vi "time wait.vi"(8 "errorIn":errorcluster, 10 "delay(s)":u32=2000, 11 "Mode?":enum16{"Light Mode", "Dark Mode"}(ring)) -> (0 "errorOut":errorcluster)   [LabVIEW 2020]
panel:
  out "Time Remaining":string="   PLEASE WAITING..."
  in  "退出":bool
  out "Cancel?":bool=TRUE
  out "Wait":string="   PLEASE WAITING..."
  out "Slide":i32(slide) scale=0.0..1800000.0
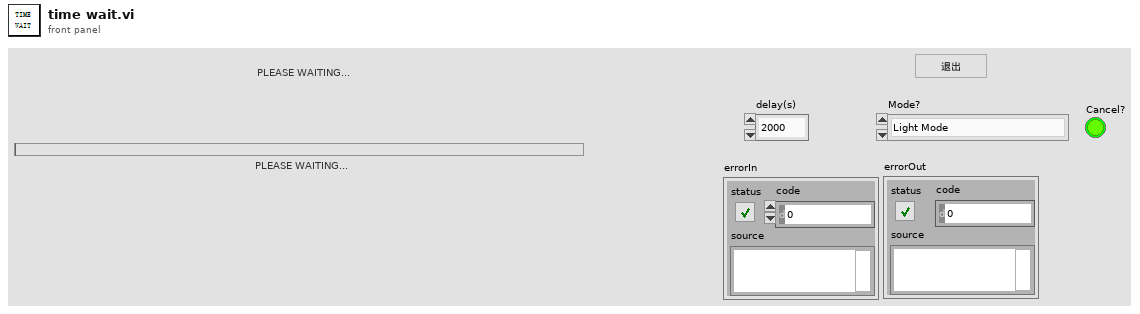
[diagram p1: front panel]
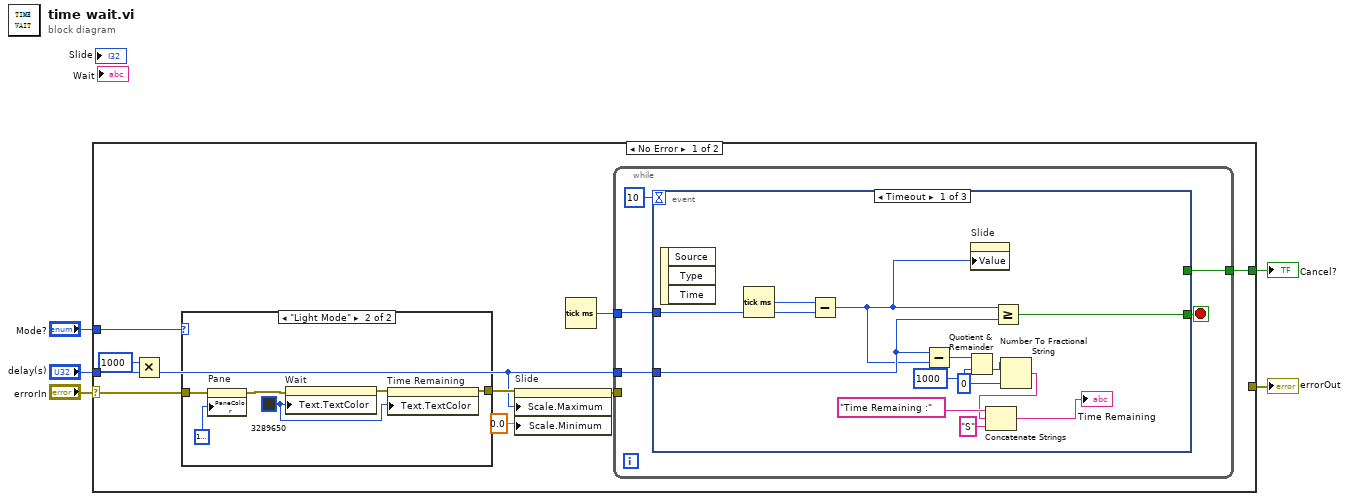
[diagram p0: block diagram]
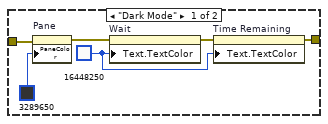
[diagram p2: hidden frame]
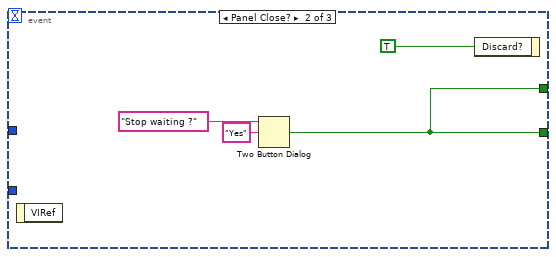
[diagram p3: hidden frame]
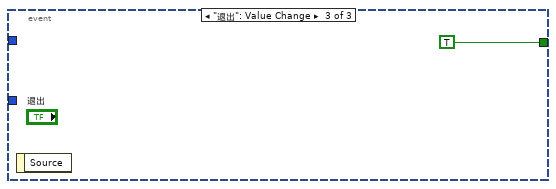
[diagram p4: hidden frame]
diagram:
  n1 = case shown="No Error" "errorIn" {
    selector: "errorIn" -> [w10 w50]
    tunnel: "delay(s)" -> [w14 _]
    tunnel: [_ w50] -> w3
    tunnel: "Mode?" -> [w11 _]
    tunnel: [w8 _] -> w1
    frame No Error {
      n2 = Multiply(x=u32 1000, y=w14) -> (x*y=w7:u32)
      n3 = case shown="\"Light Mode\"" w11 {
        tunnel: w10 -> [w20 w26]
        tunnel: [w17 w22] -> w9
        frame "Dark Mode" {
          w16 = u32 16448250
          n4 = property on="Pane" class="Pane"(error in=w20, "PaneColor"=u32 3289650) -> (error out=w18:errorcluster)  [unwired: 1 in, 1 out]
          n5 = property on="Wait" class="Str"(error in=w18, "Text.TextColor"=w16) -> (error out=w17:errorcluster)  [unwired: 1 in, 1 out]
          n6 = property on="Time Remaining" class="Str"(error in=w17, "Text.TextColor"=w16) -> ()  [unwired: 1 in, 2 out]
        }
        frame "Light Mode" {
          w21 = u32 3289650
          n7 = property on="Pane" class="Pane"(error in=w26, "PaneColor"=u32 16777238) -> (error out=w25:errorcluster)  [unwired: 1 in, 1 out]
          n8 = property on="Wait" class="Str"(error in=w25, "Text.TextColor"=w21) -> (error out=w23:errorcluster)  [unwired: 1 in, 1 out]
          n9 = property on="Time Remaining" class="Str"(error in=w23, "Text.TextColor"=w21) -> (error out=w22:errorcluster)  [unwired: 1 in, 1 out]
        }
      }
      n10 = property on="Slide" class="Slide (strict)"(error in=w9, "Scale.Maximum"=w7, "Scale.Minimum"=0.0 ("Scale.Range:Minimum")) -> (error out=w12:errorcluster)  [unwired: 1 in, 1 out]
      n11 = Tick Count (ms)() -> (millisecond timer value=w15:u32)
      n12 = while {
        tunnel: w15 -> [w31]
        tunnel: w7 -> [w30]
        tunnel: w12 -> [_]
        tunnel: [w27] -> w8
        stop <- w29 stop-if-true
        n13 = event shown="[0] Timeout" {
          selector: _ -> [_ _ _]
          dyn-events: _ -> [_ _ _]
          timeout: 10 -> [_ _ _]
          tunnel: w31 -> [w43 _ _]
          tunnel: w30 -> [w41 _ _]
          tunnel: [w42 w45 TRUE ("T button?")] -> w29
          tunnel: [_ w45 _] -> w27
          event Timeout {
            n14 = event-data() -> ()  [unwired: 1 in, 3 out]
            n15 = Tick Count (ms)() -> (millisecond timer value=w44:u32)
            n16 = Subtract(x=w44, y=w43) -> (x-y=w40:u32)
            n17 = Subtract(x=w41, y=w40) -> (x-y=w39:u32)
            n18 = Quotient & Remainder(x=w39, y=u32 1000) -> (floor(x/y)=w35:u32)  [unwired: 1 out]
            n19 = property on="Slide" class="Slide (strict)"("Value"=w40) -> ()  [unwired: 2 in, 2 out]
            n20 = Greater Or Equal?(x=w40, y=w41) -> (x >= y?=w42:bool)
            n21 = Number To Fractional String(number=w35, precision (6)=i16 0) -> (F-format string=w36:string)  [unwired: 2 in]
            n22 = Concatenate Strings("Time Remaining :" ("time remaining"), w36, "S" ("string")) -> (→"Time Remaining":string)
          }
          event Panel Close? {
            n23 = event-data() -> ()  [unwired: 1 in, 1 out]
            n24 = Two Button Dialog(message="Stop waiting ?", 2:"Yes" ("T button name (\"OK\")")) -> (T button?=w45:bool)  [unwired: 1 in]
            n25 = event-data("Discard?"=TRUE) -> ()  [unwired: 1 in, 1 out]
          }
          event "退出": Value Change {
            n26 = event-data() -> ()  [unwired: 1 in, 1 out]
          }
        }
      }
    }
    frame Error {
    }
  }
  "errorOut" <- w3
  "Cancel?" <- w1
